vi "Test Copy Image Greyscale Mask Greyscale.vi"(8 "error in (no error)":errorcluster, 11 "Test Case In":refnum<class "Image.lvclass">) -> (0 "error out":errorcluster, 3 "Test Case Out":refnum<class "Image.lvclass">)   [LabVIEW 2020, in "g_ar_toolkit.test.lvlib" / "Image.lvclass"]
uses:
  Image.lvclass
  C:/Program Files (x86)/National Instruments/LabVIEW 2020/vi.lib/Astemes/LUnit/Test Case.lvclass
  g_ar_toolkit.common/Image Size (Integer).ctl
  <vilib>/Astemes/LUnit/Test Case.lvclass/Test Case.ctl
  g_ar_toolkit.image/New Image (Greyscale).vi
  g_ar_toolkit.image/Copy Array to Image (Greyscale).vi
  g_ar_toolkit.image/Copy Image (Greyscale with Mask).vi
  4993e8ee-a06a-463a-9684-69129f64d5ce.vi
  g_ar_toolkit.image/New Image (Greyscale).vi/6598b9e0-8a08-46f5-91fd-ca1b87217137.vi
  g_ar_toolkit.image/Copy Image (Greyscale with Mask).vi/1519c485-f8d8-4564-b4f6-4c035770646f.vi
  <vilib>/Astemes/LUnit/Append Pass Result.vi
  <vilib>/Astemes/LUnit/Append Fail Result.vi
  <vilib>/Astemes/LUnit/Describe Comparison.vi
  4993e8ee-a06a-463a-9684-69129f64d5ce.vi/9c5d11cd-9439-4240-a1ee-d9baace9c924.vi
  <vilib>/Astemes/LUnit/Run In UI.vi
  <vilib>/Utility/error.llb/Clear Errors.vi
  g_ar_toolkit.common/Module Path.vi
  <vilib>/Utility/error.llb/Error Cluster From Error Code.vi
  <vilib>/picture/pixmap.llb/Flatten Pixmap.vi
  <vilib>/Astemes/LUnit/Describe Variant.vi
  Image.lvclass/Image.ctl
  g_ar_toolkit.image/g_ar_toolkit.image.lvlib
  g_ar_toolkit.common/g_ar_toolkit.common.lvlib
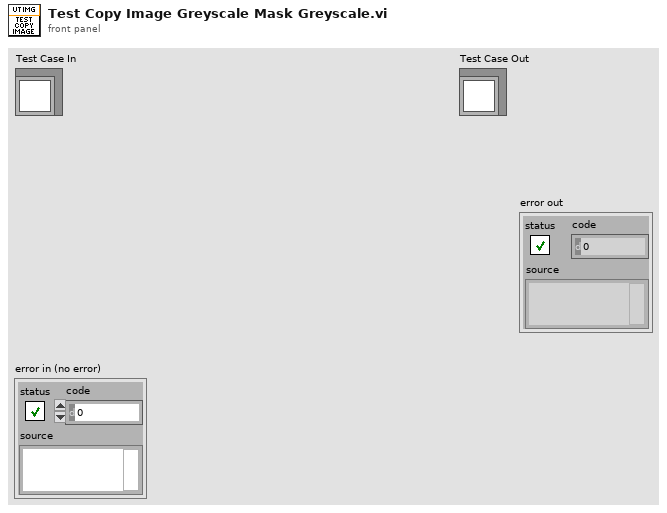
[diagram p1: front panel]
types:
  T1 = typedef "g_ar_toolkit.common.lvlib/Image Size (Integer).ctl" = cluster{"Width":u16, "Height":u16}
  T2 = typedef "g_ar_toolkit.image.lvlib/Greyscale Image.ctl" = refnum<data-value>
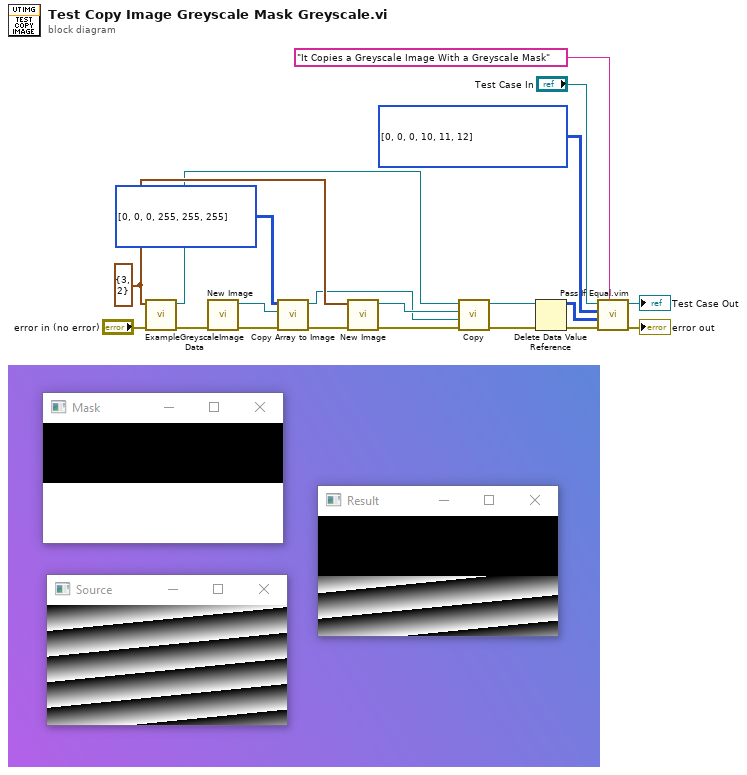
[diagram p0: block diagram]
diagram:
  w12 = T1 {"Width"=3, "Height"=2} ("Preallocated Image Size (Default - 0,0)")
  n1 = call "ExampleGreyscaleImageData.vi"("error in (no error)"="error in (no error)", "Image Size"=w12) -> ("error out"=w10:errorcluster, "Greyscale Destination Image"=w3:T2)  [unwired: 6 in, 2 out]
  n2 = call-poly "New Image.vi"("error in (no error)"=w10) -> ("error out"=w15:errorcluster, "New Greyscale Image"=w8:T2)  [unwired: 9 in]
  n3 = call-poly "Copy Array to Image.vi"("error in (no error)"=w15, "Greyscale Destination Image"=w8, "U8 Greyscale Data"=u8[][] [[0, 0, 0], [255, 255, 255]] ("Source")) -> ("error out"=w9:errorcluster, "Greyscale Destination Image (duplicate)"=w5:T2)  [unwired: 7 in]
  n4 = call-poly "New Image.vi"("error in (no error)"=w9, "Preallocated Image Size (Default 0,0)"=w12) -> ("error out"=w4:errorcluster, "New Greyscale Image"=w6:T2)  [unwired: 8 in]
  n5 = call-poly "Copy.vi"("error in (no error)"=w4, "Greyscale Image Mask"=w5, "Greyscale Image Destination"=w6, "Greyscale Image Source"=w3) -> ("error out"=w16:errorcluster, "Greyscale Image Destination (duplicate)"=w14:T2)  [unwired: 6 in]
  n6 = Delete Data Value Reference(data value reference=w14, error in=w16) -> (data value=w1:u8[][], error out=w13:errorcluster)
  n7 = call "Pass If Equal.vim"("Description"="It Copies a Greyscale Image With a Greyscale Mask", "error in (no error)"=w13, "Actual"=w1, "Expected"=u8[][] [[0, 0, 0], [10, 11, 12]] ("data value"), "LUnit Test Case In"="Test Case In") -> ("error out"=→"error out":errorcluster, "LUnit Test Case Out"=→"Test Case Out":refnum<class "Image.lvclass">)  [unwired: 5 in]
